vi "Test Fit N Gaussians.vi"() -> ()   [LabVIEW 2011]
panel:
  out "Initial Parameters":T1(array[cluster])
  in  "Standard Deviation":dbl=4.0
  in  "Kernel Size":i32=13
  out "number of function calls":i32
  out "Best-Fit Parameters":T1(array[cluster])
  out "Best Fit Image":T2(plugin-control)
  in  "Range":cluster{"Lower value":sgl, "Upper value":sgl}={"Lower value"=150.0, "Upper value"=32768.0}
  out "Image":T2(plugin-control)
  in  "stop":bool
  in  "File Path":path=path "C:/Users/Behavior Room/Dropbox/Science/Datta lab/Kinect Mouse/Kinect/Experimental/Gaussian Fitting/Proximal Mice.tiff"
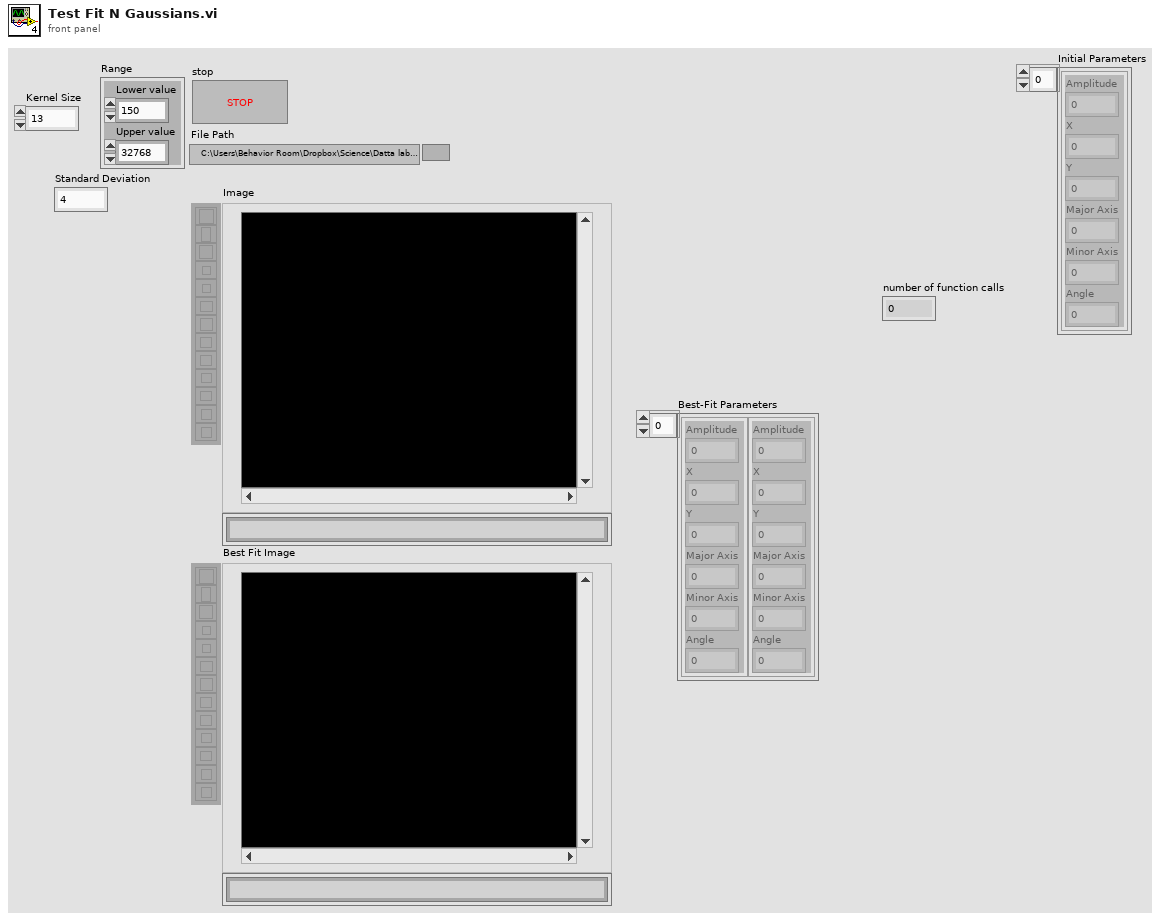
[diagram p1: front panel]
types:
  T1 = cluster{"Amplitude":dbl, "X":dbl, "Y":dbl, "Major Axis":dbl, "Minor Axis":dbl, "Angle":dbl}[]
  T2 = typedef "IMAQ Image.ctl" = refnum<image>
  T3 = typedef "Image Type" = u32
  T4 = cluster{"Area":dbl, "Number of Holes":dbl, "Bounding Rect":cluster{"Left":dbl, "Top":dbl, "Right":dbl, "Bottom":dbl}, "Center of Mass":cluster{"X":dbl, "Y":dbl}, "Orientation":dbl, "Dimensions":cluster{"Width":dbl, "Height":dbl}}[]
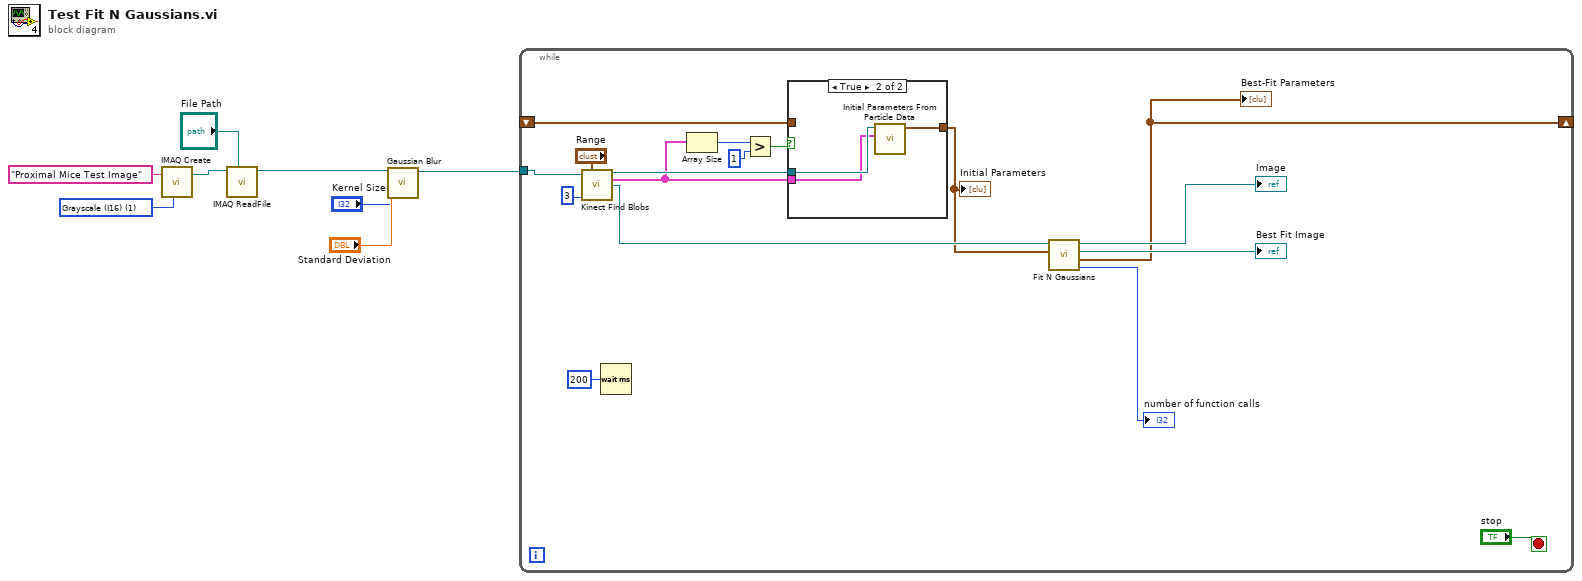
[diagram p0: block diagram]
diagram:
  w5 = T3 1 items=["Grayscale (U8)", "Grayscale (I16)", "Grayscale (SGL)", "Complex (CSG)", "RGB (U32)", "HSL (U32)", "RGB (U64)", "Grayscale (U16)"] ("Image Type")
  n1 = call "IMAQ Create"("Image Name"="Proximal Mice Test Image", "Image Type"=w5) -> ("New Image"=w7:T2)  [unwired: 3 in, 1 out]
  n2 = call "IMAQ ReadFile"("File Path"="File Path", "Image"=w7) -> ("Image Out"=w2:T2)  [unwired: 5 in, 4 out]
  n3 = call "Gaussian Blur.vi"("Standard Deviation"="Standard Deviation", "Kernel Size"="Kernel Size", "Image"=w2) -> ("Image Out"=w1:T2)  [unwired: 8 in]
  n4 = while {
    tunnel: w1 -> [w22]
    shift-right: [w14] -> _
    shift-left: _ -> [w13]
    stop <- "stop" stop-if-true
    n5 = call "Kinect Find Blobs.vi"("Image Src"=w22, "Range"="Range", "Number of Erosion"=3) -> ("Masked Image Out"=w16:T2, "Particle Reports (Pixels)"=w12:T4, "Src Image Out"=w17:T2)  [unwired: 10 in]
    n6 = Wait (ms)(milliseconds to wait=u32 200) -> ()  [unwired: 1 out]
    n7 = Array Size(array=w12) -> (size(s)=w10:i32)
    n8 = Greater?(x=w10, y=1) -> (0:w11:bool)
    n9 = case shown="True" w11 {
      tunnel: w16 -> [_ w29]
      tunnel: w12 -> [_ w28]
      tunnel: [w26 w27] -> w15
      tunnel: w13 -> [w26 _]
      frame False {
      }
      frame True {
        n10 = call "Initial Parameters From Particle Data.vi"("Particle Reports (Pixels)"=w28, "Masked Image"=w29) -> ("Array"=w27:T1)  [unwired: 9 in]
      }
    }
    "Initial Parameters" <- w15
    n11 = call "Fit N Gaussians.vi"("Initial Parameters"=w15, "Image In"=w17) -> ("number of function calls"=→"number of function calls":i32, "Best-Fit Parameters"=w14:T1, "Best-Fit Image"=→"Best Fit Image":T2, "Image Src (Original)"=→"Image":T2)  [unwired: 6 in]
    "Best-Fit Parameters" <- w14
  }
